vi "Cull and Group.vi"(8 "Min Compnt %":dbl=15.0, 9 "Score Cutoff %":dbl=70.0, 10 "Sorted Data":dbl[][](array[numeric])) -> (2 "Best Targets above cutoff":T1(array[cluster]))   [LabVIEW 2019]
doc: "Examine the particle measurements to find the most likely pair that make up the target. This primarily compares the edges of the bounding boxes. It then returns information about the best two targets, notably the rectangle sourrounding the particles and the score."
panel:
  out "Grouping Scores":T2(array[cluster])
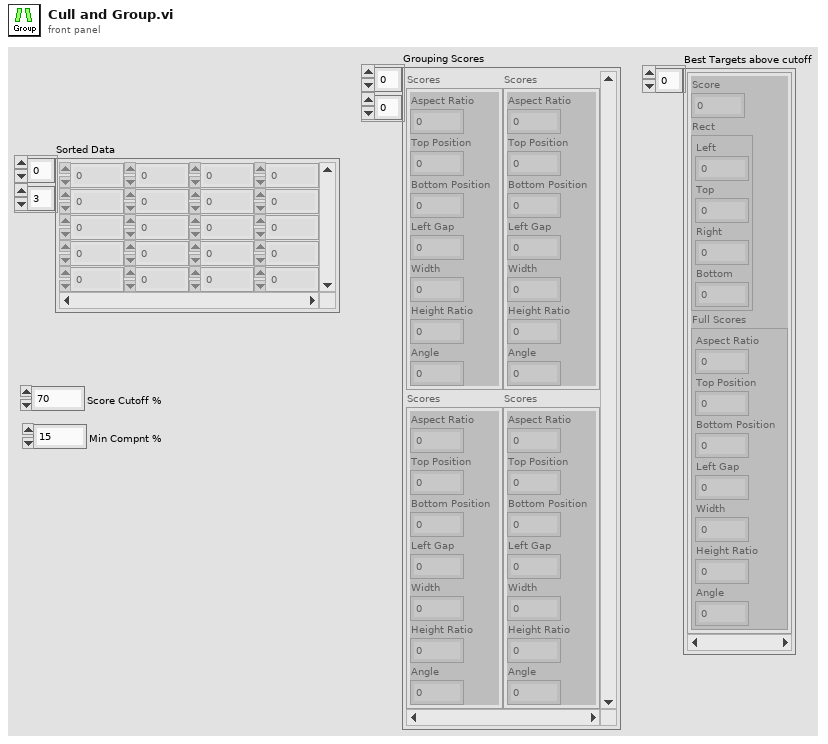
[diagram p1: front panel]
types:
  T1 = cluster{"Score":dbl, "Rect":cluster{"Left":dbl, "Top":dbl, "Right":dbl, "Bottom":dbl}, "Full Scores":cluster{"Aspect Ratio":dbl, "Top Position":dbl, "Bottom Position":dbl, "Left Gap":dbl, "Width":dbl, "Height Ratio":dbl, "Angle":dbl}}[]
  T2 = cluster{"Aspect Ratio":dbl, "Top Position":dbl, "Bottom Position":dbl, "Left Gap":dbl, "Width":dbl, "Height Ratio":dbl, "Angle":dbl}[][]
  T3 = cluster{"Left":dbl, "Top":dbl, "Right":dbl, "Bottom":dbl}
  T4 = cluster{"Aspect Ratio":dbl, "Strip Width":dbl, "Bottom Position":dbl, "Left Gap":dbl, "Width":dbl, "Height Ratio":dbl, "Angle":dbl}
  T5 = cluster{dbl, "Rect":cluster{"Left":dbl, "Top":dbl, "Right":dbl, "Bottom":dbl}, "Scores":cluster{"Aspect Ratio":dbl, "Strip Width":dbl, "Bottom Position":dbl, "Left Gap":dbl, "Width":dbl, "Height Ratio":dbl, "Angle":dbl}}
  T6 = cluster{dbl, "Rect":cluster{"Left":dbl, "Top":dbl, "Right":dbl, "Bottom":dbl}, "Scores":cluster{"Aspect Ratio":dbl, "Strip Width":dbl, "Bottom Position":dbl, "Left Gap":dbl, "Width":dbl, "Height Ratio":dbl, "Angle":dbl}}[]
  T7 = cluster{"Aspect Ratio":bool, "Strip Width":bool, "Bottom Position":bool, "Left Gap":bool, "Width":bool, "Height Ratio":bool, "Angle":bool}
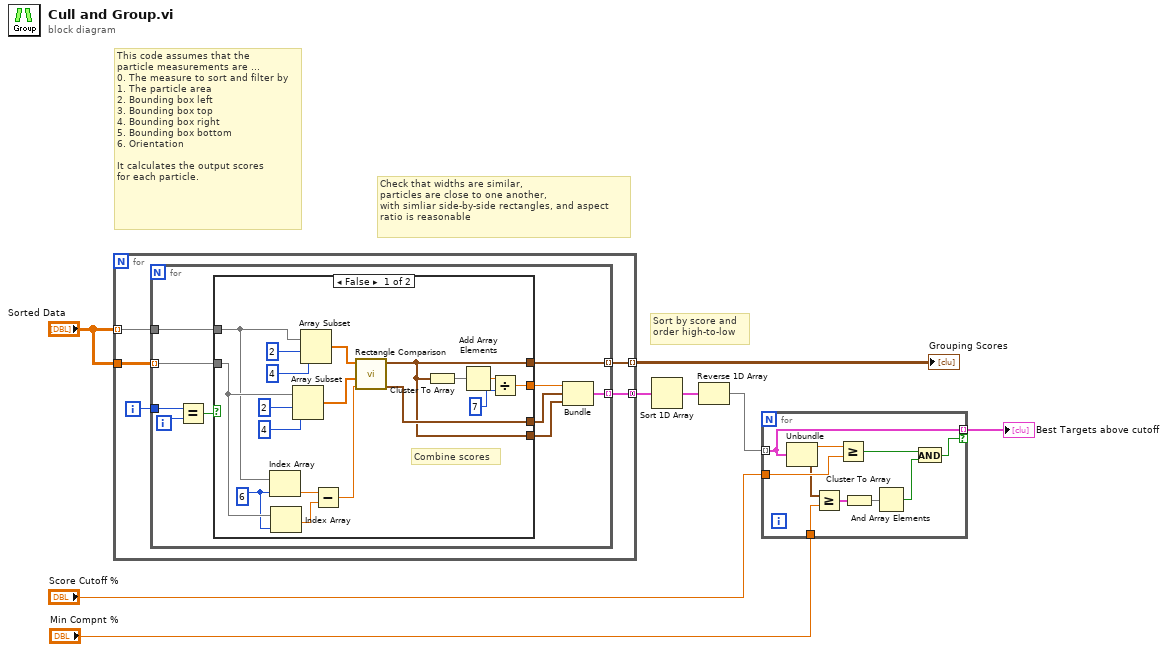
[diagram p0: block diagram]
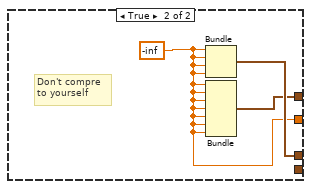
[diagram p2: hidden frame]
diagram:
  # "Sort by score and\norder high-to-low"
  # "Check that widths are similar,\nparticles are close to one another,\nwith simliar side-by-side rectangles, and aspect\nratio is reasonable"
  # "This code assumes that the\nparticle measurements are ...\n0. The measure to sort and filter by\n1. The particle area\n2. Bounding box left\n3. Bounding box top\n4. Bounding box right\n5. Bounding box bottom\n6. Orientation\n\nIt calculates the output scores\nfor each particle."
  n1 = for {
    tunnel: "Sorted Data" -> [w13] mode=indexing
    tunnel: "Sorted Data" -> [w12]
    tunnel: [w11] -> w8 mode=indexing
    tunnel: [w9] -> w6 mode=concatenating
    i -> [w10]
    n2 = for {
      tunnel: w13 -> [w23]
      tunnel: w12 -> [w21] mode=indexing
      tunnel: [w20] -> w11 mode=indexing
      tunnel: w10 -> [w19]
      tunnel: [w15] -> w9 mode=indexing
      i -> [w18]
      n3 = Equal?(x=w19, y=w18) -> (x = y?=w22:bool)
      n4 = case shown="False" w22 {
        tunnel: w23 -> [w28 _]
        tunnel: w21 -> [w29 _]
        tunnel: [w30 w43] -> w20
        tunnel: [w31 w42] -> w17
        tunnel: [w34 w44] -> w16
        tunnel: [w30 _] -> w14
        frame False {
          w27 = 6 ("index")
          # "Combine scores"
          n5 = Index Array(array=w28, index=w27) -> (element=w26:dbl)
          n6 = Index Array(array=w29, index=w27) -> (element=w25:dbl)
          n7 = Array Subset(array=w29, index=2, length=4) -> (w35:dbl[])
          n8 = Array Subset(array=w28, index=2, length=4) -> (w36:dbl[])
          n9 = Subtract(x=w26, y=w25) -> (x-y=w24:dbl)
          n10 = call "Rectangle Comparison.vi"("Angle (deg)"=w24, "Second"=w35, "First"=w36) -> ("Rect"=w34:T3, "Scores"=w30:T4)  [unwired: 7 in]
          n11 = Cluster To Array(cluster=w30) -> (array=w37:dbl[])
          n12 = Add Array Elements(numeric array=w37) -> (sum=w32:dbl)
          n13 = Divide(x=w32, y=7 ("length")) -> (x/y=w31:dbl)
        }
        frame True {
          w42 = -inf
          # "Don't compre\nto yourself"
          n14 = Bundle(w42, w42, w42, w42) -> (w44:cluster{dbl, dbl, dbl, dbl})  [unwired: 1 in]
          n15 = Bundle(w42, w42, w42, w42, w42, w42, w42) -> (w43:cluster{dbl, dbl, dbl, dbl, dbl, dbl, dbl})  [unwired: 1 in]
        }
      }
      n16 = Bundle(w17, "Rect"=w16, "Scores"=w14) -> (w15:T5)  [unwired: 1 in]
    }
  }
  "Grouping Scores" <- w8
  n17 = Sort 1D Array(array=w6) -> (sorted array=w5:T6)
  n18 = Reverse 1D Array(array=w5) -> (reversed array=w4:T6)
  n19 = for {
    tunnel: w4 -> [w54] mode=indexing
    tunnel: [w54] -> w2 mode=indexing if=w45
    tunnel: "Score Cutoff %" -> [w52]
    tunnel: "Min Compnt %" -> [w50]
    n20 = Unbundle(w54) -> (w53:dbl, "Scores"=w51:T4)  [unwired: 1 out]
    n21 = Greater Or Equal?(x=w51, y=w50) -> (x >= y?=w49:T7)
    n22 = Greater Or Equal?(x=w53, y=w52) -> (x >= y?=w46:bool)
    n23 = Cluster To Array(cluster=w49) -> (array=w48:bool[])
    n24 = And Array Elements(Boolean array=w48) -> (logical AND=w47:bool)
    n25 = And(x=w46, y=w47) -> (x .and. y?=w45:bool)
  }
  "Best Targets above cutoff" <- w2
